vi "Thermometer.vi"() -> ()   [LabVIEW 2018]
doc: "This VI acquires temperature data one value at a time from a simulateion. It scales the temperature and displays it ins a thermometer."
panel:
  out "Temperature (deg F)":dbl
  out "Reading (deg C))":dbl(slide) scale=0.0..100.0
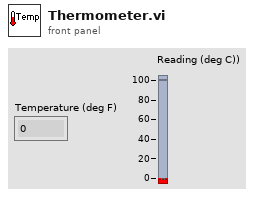
[diagram p1: front panel]
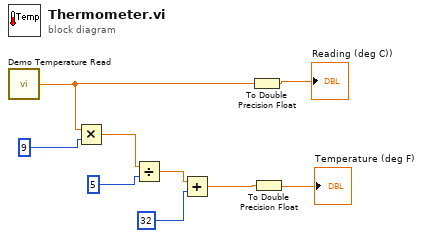
[diagram p0: block diagram]
diagram:
  n1 = call "Demo Temperature Read.vi"() -> ("Measured Temperature (degC)"=w4:dbl)  [unwired: 2 in]
  n2 = Multiply(x=w4, y=9) -> (x*y=w5:dbl)
  n3 = Divide(x=w5, y=5) -> (x/y=w6:dbl)
  n4 = Add(x=w6, y=32) -> (x+y=w3:dbl)
  n5 = To Double Precision Float(number=w4) -> (double precision float=→"Reading (deg C))":dbl)
  n6 = To Double Precision Float(number=w3) -> (double precision float=→"Temperature (deg F)":dbl)
